vi "Sequence Globals.vi"() -> ()   [LabVIEW 2018]
panel:
  out "DevSupportPath":path
  out "CalPopupTimer File":path
  out "AppSupportPath 3":path
  out "AppSupportPath 2":path
  out "AppSupportPath":path
  out "IsRuntime?":bool
  out "Gitlog":string="#RageATE gitlog: commit 3f967c02fb9022fedaa326db1cba8dee33b37288\n#RageATE gitlog: Author: Rick-Rage <74794943+Rick-Rage@users.noreply.github.com>\n#RageATE gitlog: Date:   Tue Nov 23 14:33:10 2021 -0500\n#RageATE gitlog: This Computer Name : CRANES\r\n\r\n"
  out "RageATE_Gitlog":string="#RageATE gitlog: commit 3f967c02fb9022fedaa326db1cba8dee33b37288\n#RageATE gitlog: Author: Rick-Rage <74794943+Rick-Rage@users.noreply.github.com>\n#RageATE gitlog: Date:   Tue Nov 23 14:33:10 2021 -0500\n#RageATE gitlog: This Computer Name : CRANES\r\n\r\n"
  out "Current Iteration":i32=1
  out "Inst File":path
  out "Calibration File Name":path
  out "Payload Name":string
  out "Sequence Result Directory":path
  in  "Stop Testing":bool
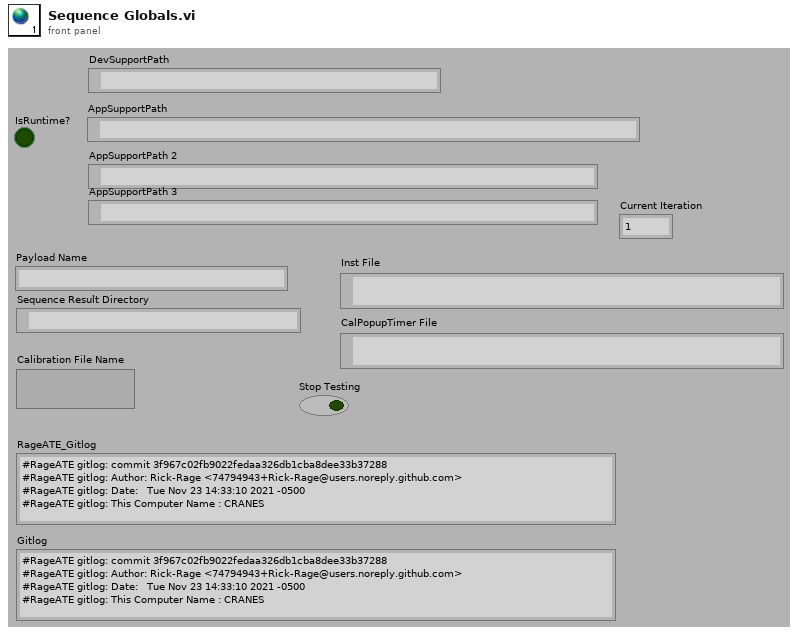
[diagram p1: front panel]
diagram:
